vi "Light_Create.vi"(0 "reference in":refnum<class "Light.lvclass">, 5 "Error In":errorcluster) -> (14 "reference out":refnum<class "Light.lvclass">, 19 "Error Out":errorcluster)   [LabVIEW 2024, in "Light.lvclass"]
uses:
  Light.lvclass/Light.ctl
  Light.lvclass
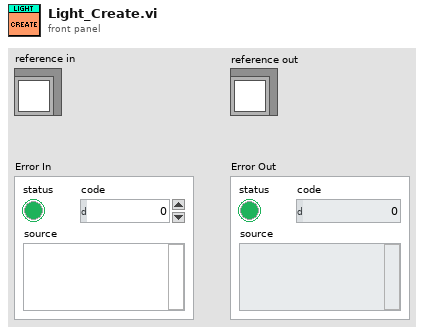
[diagram p1: front panel]
types:
  T1 = typedef "Light.lvclass/ObjectAttributes.ctl" = cluster{"State":bool}
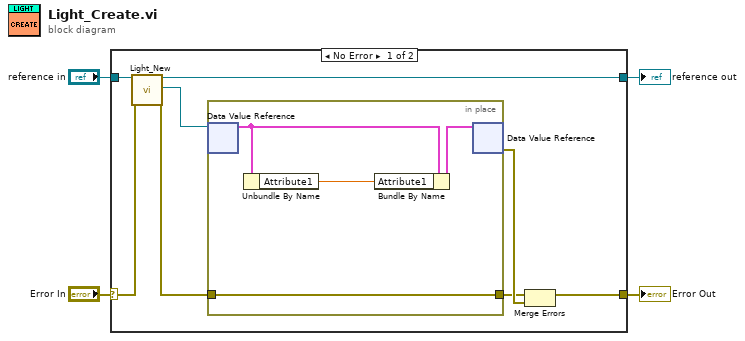
[diagram p0: block diagram]
diagram:
  n1 = case shown="No Error" "Error In" {
    selector: "Error In" -> [w11 w18]
    tunnel: [w8 w18] -> w3
    tunnel: "reference in" -> [w12 w17]
    tunnel: [w10 w17] -> w1
    frame No Error {
      n2 = call "Light_New.vi"("reference in"=w12, "Error In"=w11) -> ("reference out"=w10:refnum<class "Light.lvclass">, "DVRRefOut"=w7:refnum<data-value>, "Error Out"=w6:errorcluster)  [unwired: 14 in, 1 out]
      n3 = in-place {
        in-place-border: w6 -> [w13]
        in-place-border: [w13] -> w5
        n4 = in-place-dvr #1(w7) -> (w15:T1)  [unwired: 1 out]
        n5 = Unbundle By Name(w15) -> ("Attribute1"=w14:dbl)
        n6 = Bundle By Name(cluster=w15, "Attribute1"=w14) -> (w16:T1)
        n7 = in-place-dvr #1(w16) -> (w9:errorcluster)  [unwired: 1 out]
      }
      n8 = Merge Errors(w5, w9) -> (w8:errorcluster)
    }
    frame Error {
      # "VI-TechBaseTemplate_Simple_6x8x6"
    }
  }
  "Error Out" <- w3
  "reference out" <- w1
